vi "Read All Values.vi"(8 "error in (no error)":errorcluster, 11 "Current Value Table":T1) -> (0 "error out":errorcluster, 1 "Values":variant[](array[variant]), 2 "Names":string[](array[string]), 3 "Current Value Table":T1)   [LabVIEW 2015, in "CurrentValueTable.lvlib" / "CurrentValueTable.lvclass"]
uses:
  CurrentValueTable.lvclass
  CurrentValueTable Reference.ctl
  CurrentValueTable.lvclass/CurrentValueTable.ctl
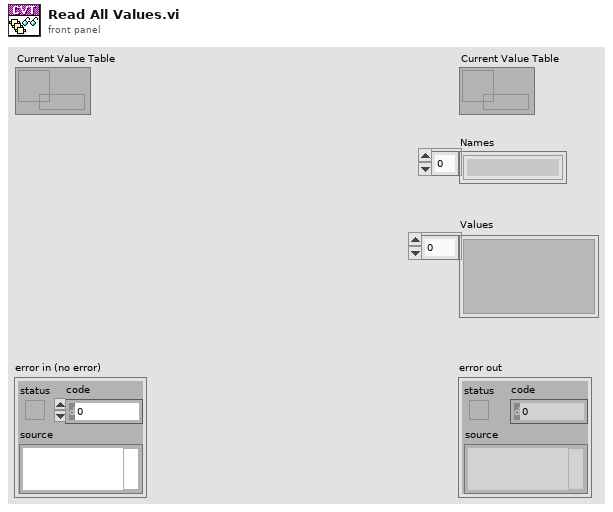
[diagram p1: front panel]
types:
  T1 = typedef "CurrentValueTable.lvlib/CurrentValueTable.lvclass/CurrentValueTable Reference.ctl" = refnum<data-value>
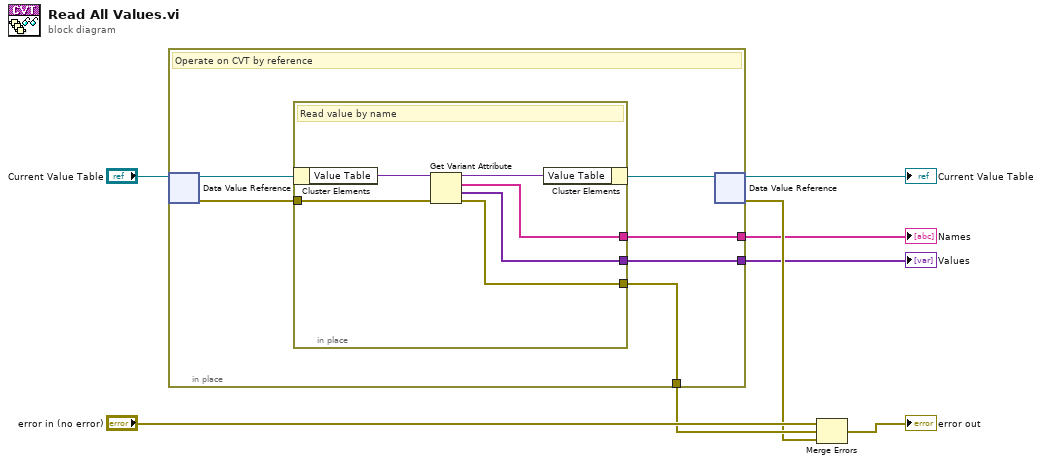
[diagram p0: block diagram]
diagram:
  n1 = in-place {
    in-place-border: [w11] -> w4
    in-place-border: [w14] -> w2
    in-place-border: [w9] -> w1
    # "Operate on CVT by reference"
    n2 = in-place-dvr #1("Current Value Table") -> (w13:refnum<class "CurrentValueTable.lvclass">, w10:errorcluster)
    n3 = in-place {
      in-place-border: w10 -> [w20]
      in-place-border: [w19] -> w11
      in-place-border: [w16] -> w14
      in-place-border: [w15] -> w9
      # "Read value by name"
      n4 = in-place-cluster #2(w13) -> ("Value Table"=w18:variant)
      n5 = Get Variant Attribute(Variant=w18, error in=w20) -> (duplicate Variant=w17:variant, names=w15:string[], values=w16:variant[], error out=w19:errorcluster)  [unwired: 2 in]
      n6 = in-place-cluster #2("Value Table"=w17) -> (w12:refnum<class "CurrentValueTable.lvclass">)
    }
    n7 = in-place-dvr #1(w12) -> (→"Current Value Table":T1, w3:errorcluster)
  }
  "Values" <- w2
  "Names" <- w1
  n8 = Merge Errors("error in (no error)", w4, w3) -> (→"error out":errorcluster)
